vi "2_PatchCore_Inference(Image).vi"() -> ()   [LabVIEW 2020]
uses:
  PatchCore_AddOn/API/Controls/NN_Paths.ctl
  PatchCore_AddOn/API/Controls/PatchCore_Init_Custom_NN_CFG.ctl
  <vilib>/Ngene/Deep Learning Toolkit/Toolkit/NN_Data/API/NN_Dims(C,H,W).ctl
  <vilib>/Ngene/Deep Learning Toolkit/Toolkit/NN_Network/Controls/NN_Device.ctl
  PatchCore_AddOn/API/Controls/Heatmap_Config.ctl
  PatchCore_AddOn/API/Controls/ColorMap.ctl
  PatchCore_AddOn/API/Controls/Feature_Scorer_Params.ctl
  PatchCore_AddOn/API/Controls/Gaussian_Blur.ctl
  PatchCore_AddOn/API/Controls/PCore_Device.ctl
  <vilib>/Utility/miscctls.llb/LVMinMaxIncTypeDef.ctl
  subVIs/Dataset_Reader/Controls/ImRead_PreProcessing_Options.ctl
  PatchCore_AddOn/Low_Level/Controls/Normalization_Type.ctl
  PatchCore_AddOn/API/NNPC_Predict/NNPC_Predict(Single).vi
  PatchCore_AddOn/PatchCore_AddOn.lvlib
  <vilib>/Ngene/Deep Learning Toolkit/Toolkit/Deep_Learning_Toolkit_by_Ngene.lvlib
panel:
  in  "PCore_Device":T1=enum."GPU(CuLab)"
  out "Image_Thrshld (Eval)":sgl=1.3846
  in  "Image_Thrshld(Custom)":sgl=-1.0 format="%_5g"
  out "dT_Predict":dbl=0.00989810000001512 format="%#_3ps"
  out "Pixel_Score(Min)":sgl=0.030176789
  out "Pixel_Score(Max)":sgl=2.5852501
  out "Image_File_Path":path=path "D:/MVTec/bottle/test/broken_large/011.png"
  in  "Feature_Scorer_Params":T2={"Nearest_Neihbours"=1, "Calculate Anomaly Map"=TRUE, "Gaussian_Blur"={"Kernel_Size"=33, "sigma"=4.0}}
  out "Pixel_Thrshld (Eval)":sgl=1.2317
  in  "Report_Image_Dims":cluster{"X Resolution":i32, "Y Resolution":i32}={"X Resolution"=224, "Y Resolution"=224}
  in  "Stop":bool
  in  "Heatmap_Config":T4={"ColorMap_Type"=enum."Jet", "Alpha"=0.4}
  out "Anomaly?":bool=TRUE
  in  "Eval_Stats_File_Path":path=path "D:/Ngene/GitHub/3_Image_Processing/36_Anomaly_Detection/Models/Patchcore_Models/__24_10_30__20_44_16/PatchCore_Eval_Stats__24_10_30__20_47_45.cfg"
  out "dT_ImRead":dbl=0.02204290000000242 format="%#_4ps"
  in  "NNFE_Custom_CFG":T6={"Input3D_Custom_Dims"={"C"=-1, "H"=-1, "W"=-1}, "mBatch"=1, "NN_Device"=enum."GPU"}
  in  "PatchCore_Paths":T9={"CFG"=path "D:/Ngene/GitHub/3_Image_Processing/36_Anomaly_Detection/Models/Patchcore_Models/__24_10_30__20_44_16/PatchCore_Config.cfg", "BIN"=path "D:/Ngene/GitHub/3_Image_Processing/36_Anomaly_Detection/Models/Patchcore_Models/__24_10_30__20_44_16/MemBank_NNFE_WRN_50_2_L2L3_PS3_RP296_SR0.1_Size16.4k.bin"}
  in  "NNFE_Paths":T9={"CFG"=path "D:/Ngene/GitHub/3_Image_Processing/36_Anomaly_Detection/Models/Patchcore_Models/__24_10_30__20_44_16/NNFE_WRN_50_2_L2L3_PS3_RP296.cfg", "BIN"=path "D:/Ngene/GitHub/3_Image_Processing/36_Anomaly_Detection/Models/Patchcore_Models/__24_10_30__20_44_16/NNFE_WRN_50_2_L2L3_PS3_RP296.bin"}
  out "Anomaly Detection Results":T10(plugin-control)
  out "Img_Score":sgl=2.7060041
  in  "Image_idx":u32=31 max=82
  in  "Ground_Truth_Folder_Path":path=path "D:/MVTec/bottle/ground_truth"
  in  "Pixel_Thrshld(Custom)":sgl=-1.0 format="%_5g"
  in  "Test_Dataset_Folder_Path":path=path "D:/MVTec/bottle/test"
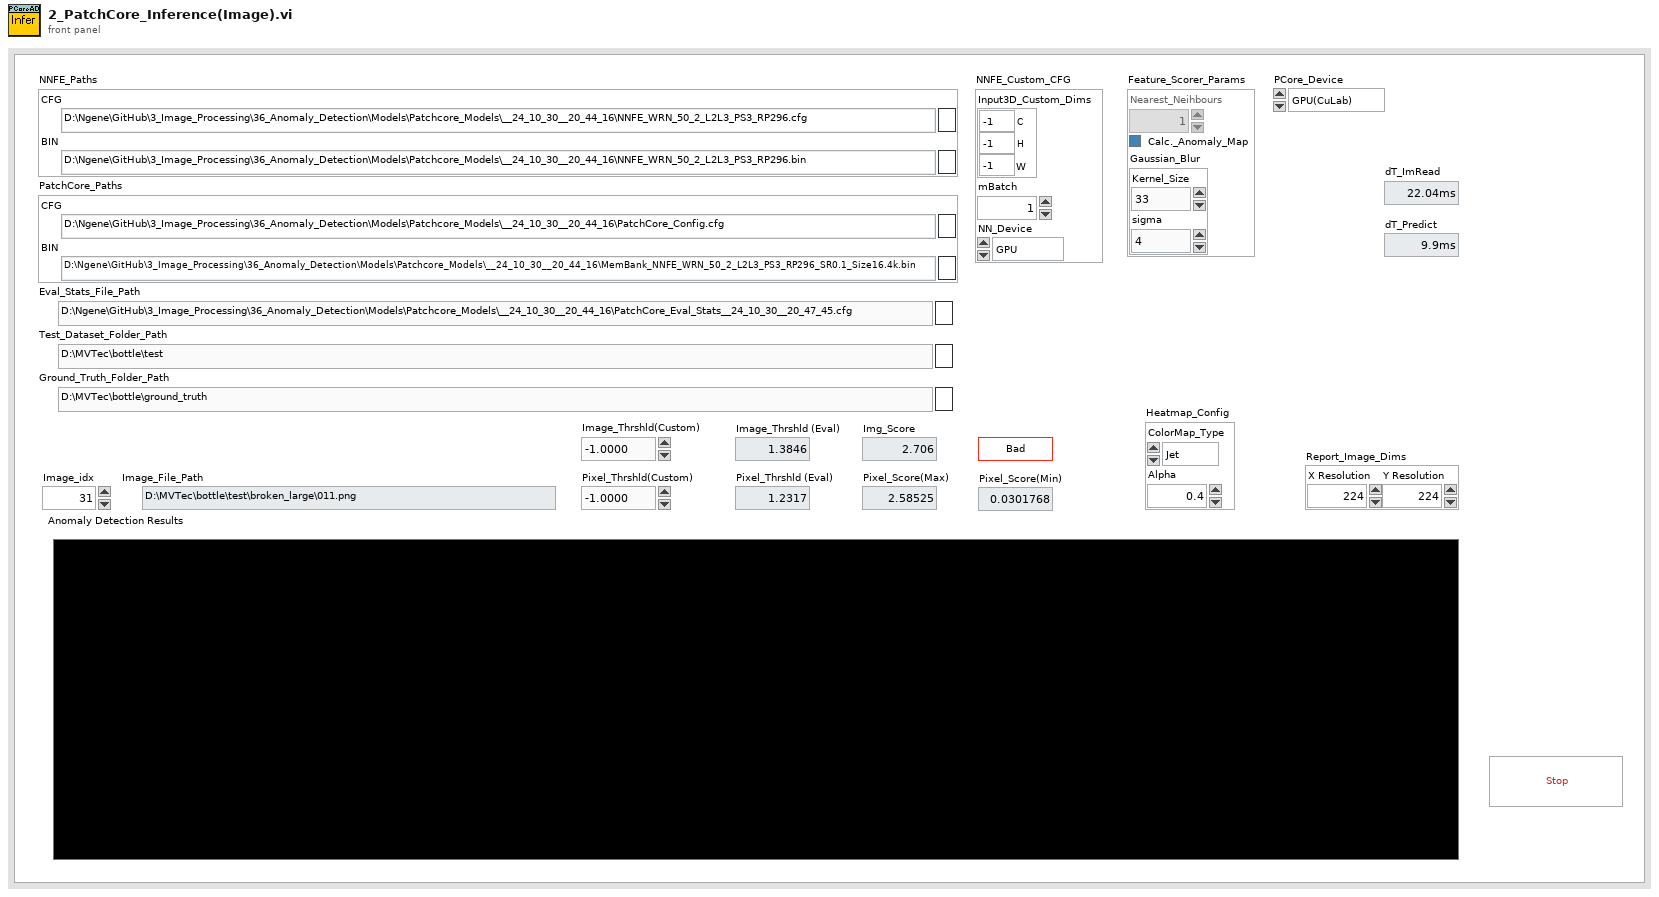
[diagram p1: front panel]
types:
  T1 = typedef "PatchCore_AddOn.lvlib/PCore_Device.ctl" = enum16{"CPU", "GPU(CuLab)"}
  T2 = typedef "PatchCore_AddOn.lvlib/Feature_Scorer_Params.ctl" = cluster{"Nearest_Neihbours":i32, "Calculate Anomaly Map":bool, "Gaussian_Blur":T3}
  T3 = typedef "PatchCore_AddOn.lvlib/Gaussian_Blur.ctl" = cluster{"Kernel_Size":i32, "sigma":sgl}
  T4 = typedef "PatchCore_AddOn.lvlib/Heatmap_Config.ctl" = cluster{"ColorMap_Type":T5, "Alpha":sgl}
  T5 = typedef "PatchCore_AddOn.lvlib/ColorMap.ctl" = enum16{"Jet", "Perula", "Inferno", "Plasma", "Viridis"}
  T6 = typedef "PatchCore_AddOn.lvlib/PatchCore_Init_Custom_NN_CFG.ctl" = cluster{"Input3D_Custom_Dims":T7, "mBatch":i32, "NN_Device":T8}
  T7 = typedef "Deep_Learning_Toolkit_by_Ngene.lvlib/NN_Dims(C,H,W).ctl" = cluster{"C":i32, "H":i32, "W":i32}
  T8 = typedef "Deep_Learning_Toolkit_by_Ngene.lvlib/NN_Device.ctl" = enum16{"CPU", "GPU"}
  T9 = typedef "PatchCore_AddOn.lvlib/NN_Paths.ctl" = cluster{"CFG":path, "BIN":path}
  T10 = typedef "IMAQ Image.ctl" = refnum<image>
  T11 = typedef "LVMinMaxIncTypeDef.ctl" = cluster{"Minimum":dbl, "Maximum":dbl, "Increment":dbl}
  T12 = typedef "PatchCore_AddOn.lvlib/PatchCore_Instance.ctl" = cluster{"Dataset_Stats":T13, "NN":T15, "PCore_Device":T1, "PatchCore_Init_CFG":T30, "Coreset Params":T32, "MemBank_Data":T34}
  T13 = typedef "PatchCore_AddOn.lvlib/PatchCore_DS_Stats.ctl" = cluster{"means":T14, "vars":T14, "DS_Size":i32}
  T14 = typedef "PatchCore_AddOn.lvlib/Image_Stats_RGB.ctl" = cluster{"R":sgl, "G":sgl, "B":sgl}
  T15 = typedef "Deep_Learning_Toolkit_by_Ngene.lvlib/NN.ctl" = cluster{"Name":string, "No of Layers":i32, "mBatch":i32, "Layers":T16[], "Dimty":T17, "Dims_In":T7, "Dims_Out":T7, "Working_Dir":path, "Train?":bool, "Train_Params":T18, "LR_Update_Policy":T21, "Session Data":T23, "Ground_truth":T24, "NNg_hdls":T25, "NN_Device":T8, "GPU Id":i32, "Labels":string[], "Receptive Field":T26[], "Loss_Type":T27, "Loss_Cfg_Prms":variant, "NNG_WS":T28}
  T16 = typedef "Deep_Learning_Toolkit_by_Ngene.lvlib/NN_Layer_ref.ctl" = refnum<data-value>
  T17 = typedef "Deep_Learning_Toolkit_by_Ngene.lvlib/NN_In_Out_Dim-ty.ctl" = enum8{"In1D_Out1D", "In3D_Out1D", "In3D_Out3D", "In3D_OutBBox"}
  T18 = typedef "Deep_Learning_Toolkit_by_Ngene.lvlib/NN_Train_Params.ctl" = cluster{"Optimizer":T19, "Beta_1":sgl, "Beta_2":sgl, "Weight Decay(L1)":sgl, "Weight Decay(L2)":sgl, "Data_Sampling":T20}
  T19 = typedef "Deep_Learning_Toolkit_by_Ngene.lvlib/NN_Train_Optimizer.ctl" = enum16{"SGD", "Adam", "Adagrad", "Adadelta", "RMSProp", "Nesterov"}
  T20 = typedef "Deep_Learning_Toolkit_by_Ngene.lvlib/NN_Train_Data_Sampling.ctl" = enum16{"Random", "Sequential"}
  T21 = typedef "Deep_Learning_Toolkit_by_Ngene.lvlib/NN_LR_Policy_Cfg.ctl" = cluster{"Policy_Type":T22, "LR0":dbl, "k":sgl, "WarmUp_Policy":enum16{"Step", "Ramp"}, "WarmUp_Iter":i32, "WarmUp_Ratio":sgl}
  T22 = typedef "Deep_Learning_Toolkit_by_Ngene.lvlib/NN_LR_Policy_Type.ctl" = enum16{"Manual", "Step", "Exp", "1/t"}
  T23 = typedef "Deep_Learning_Toolkit_by_Ngene.lvlib/NN_Train_Session_Data.ctl" = cluster{"Epochs":sgl, "Tot_Iter":i32, "LR":sgl, "LR_iter":i32}
  T24 = typedef "Deep_Learning_Toolkit_by_Ngene.lvlib/NN_Ground_truth.ctl" = cluster{"Y":variant}
  T25 = typedef "Deep_Learning_Toolkit_by_Ngene.lvlib/nng_cuda_handles.ctl" = cluster{"cudnn":u64, "cublas":u64, "stream":u64, "curand":u64}
  T26 = typedef "Deep_Learning_Toolkit_by_Ngene.lvlib/NN_Dims(V,H).ctl" = cluster{"V":i32, "H":i32}
  T27 = typedef "Deep_Learning_Toolkit_by_Ngene.lvlib/NN_Loss_Type.ctl" = enum16{"None", "MSE", "CrossEntropy", "YOLO_v2", "YOLO_v4"}
  T28 = typedef "Deep_Learning_Toolkit_by_Ngene.lvlib/NNG_WS.ctl" = cluster{"NNG_WS_Mem":T29, "Max_WS_Size":i64}
  T29 = typedef "Deep_Learning_Toolkit_by_Ngene.lvlib/NNg_WS_Mem_DVR.ctl" = refnum<data-value>
  T30 = typedef "PatchCore_AddOn.lvlib/PatchCore_Init_CFG.ctl" = cluster{"BackBone":T31, "Out_Layers_Names":string[], "Patch_Size":u32}
  T31 = typedef "PatchCore_AddOn.lvlib/PatchCore_BackBone_Selector.ctl" = enum16{"WRN_50_2_L2L3"}
  T32 = typedef "PatchCore_AddOn.lvlib/Coreset_Params.ctl" = cluster{"Sampling_Ratio":sgl, "Startd_idx":i32, "Random_Proj?":bool, "Rnd. Proj. Params":T33}
  T33 = typedef "PatchCore_AddOn.lvlib/Random_Projection_Coreset.ctl" = cluster{"Proj._Dim.":i32, "Epsilon":sgl, "Seed":i32}
  T34 = typedef "PatchCore_AddOn.lvlib/MemBank_and_Norm_Variants.ctl" = cluster{"MemBank":variant, "MemBank Norm":variant}
  T35 = typedef "PatchCore_AddOn.lvlib/Eval_Results.ctl" = cluster{"Scores(Good)":T36, "Scores(Bad)":T36, "F1_Max":sgl, "Thrshld(F1_Max)":sgl, "IoU_Max":sgl, "Thrshld(IoU_Max)":sgl, "AUROC":sgl}
  T36 = typedef "PatchCore_AddOn.lvlib/MinMax.ctl" = cluster{"Min":sgl, "Max":sgl}
  T37 = typedef "ImRead_PreProcessing_Options.ctl" = cluster{"Image Type":T38, "Normalization Type":T39, "Interpolation Type":u32}
  T38 = typedef "Image Type" = u32
  T39 = typedef "PatchCore_AddOn.lvlib/Normalization_Type.ctl" = enum16{"Standardize(DS_Stats)", "Standardize(Image_Stats)"}
  T40 = typedef "PatchCore_AddOn.lvlib/Anomaly_Detection_Results_Imgs.ctl" = cluster{"Image":T10, "Ground Truth":T10, "Predicted Heat Map":T10, "Predicted Mask":T10, "Segmentation":T10}
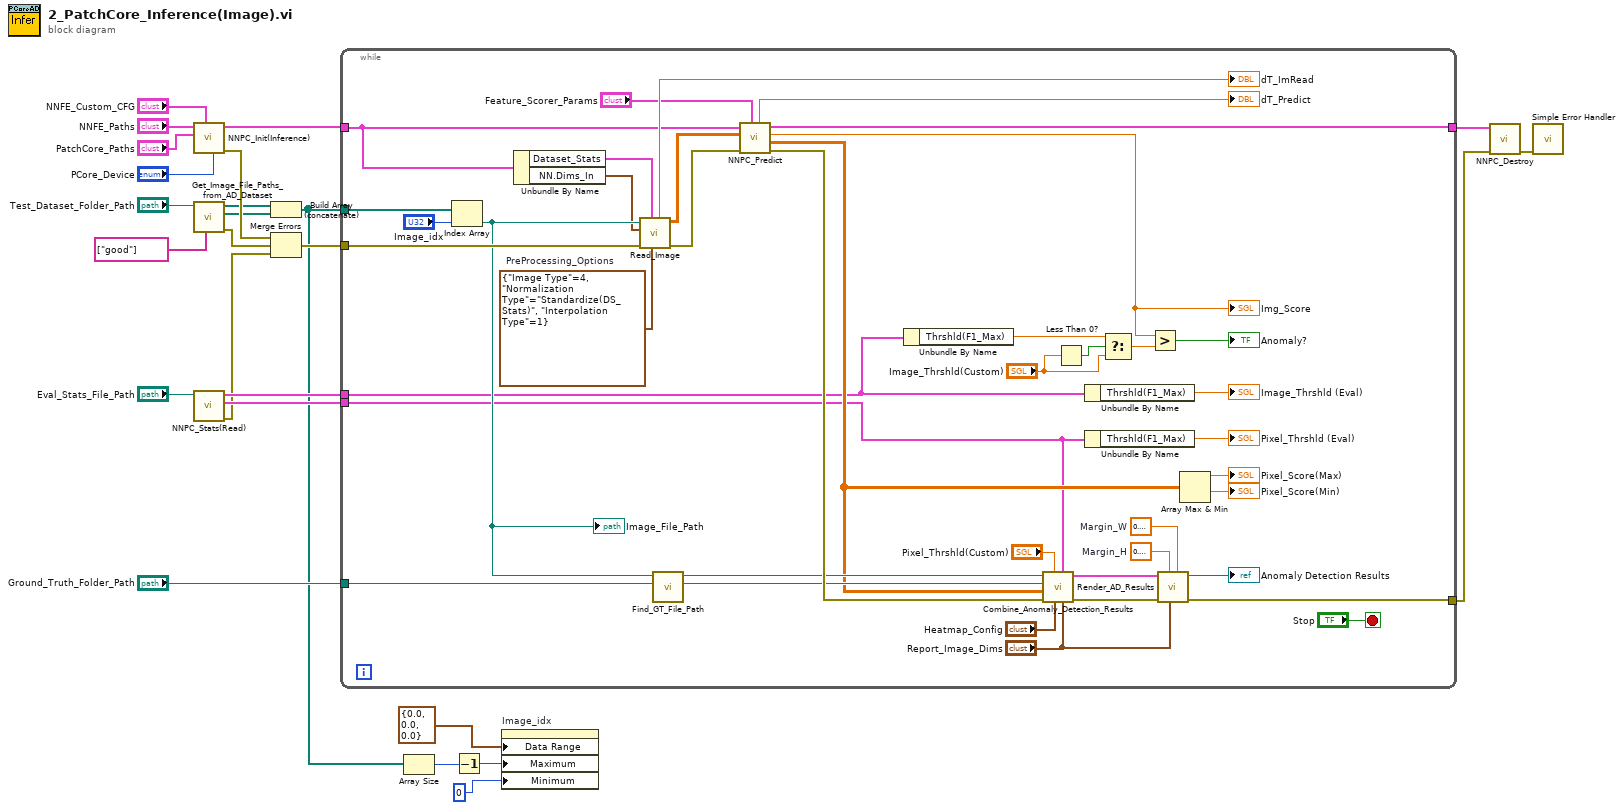
[diagram p0: block diagram]
diagram:
  n1 = call "NNPC_Init(Inference).vi"("PCore_Device"="PCore_Device", "NNFE_Custom_CFG"="NNFE_Custom_CFG", "PatchCore_Paths"="PatchCore_Paths", "NNFE_Paths"="NNFE_Paths") -> ("error out"=w14:errorcluster, "PCore_Instance out"=w19:T12)  [unwired: 6 in]
  n2 = call "Get_Image_File_Paths_from_AD_Dataset.vi"("Good Folder Names"=string[] ["good"] ("Good Folder Name"), "Dataset Folder"="Test_Dataset_Folder_Path") -> ("error out"=w9:errorcluster, "Bad Dataset Files"=w2:path[], "Good Dataset Files"=w1:path[])  [unwired: 7 in]
  n3 = call "NNPC_Stats(Read).vi"("CFG file path"="Eval_Stats_File_Path") -> ("error out"=w13:errorcluster, "Pixel Results"=w15:T35, "Image Results"=w16:T35)  [unwired: 8 in]
  n4 = Build Array (concatenate)(w1, w2) -> (w10:path[])
  n5 = Merge Errors(w14, w9, w13) -> (w17:errorcluster)
  n6 = while {
    tunnel: w10 -> [w66]
    tunnel: w19 -> [w41]
    tunnel: [w64] -> w7
    tunnel: w16 -> [w33]
    tunnel: w15 -> [w32]
    tunnel: w17 -> [w65]
    tunnel: [w60] -> w8
    tunnel: "Ground_Truth_Folder_Path" -> [w44]
    stop <- "Stop" stop-if-true
    w26 = T37 {"Image Type"=4, "Normalization Type"=enum."Standardize(DS_Stats)", "Interpolation Type"=1}  # PreProcessing_Options
    w54 = sgl 0.2  # Margin_W
    w55 = sgl 0.2  # Margin_H
    n7 = Index Array(array=w66, index="Image_idx") -> (element=w47:path)
    "Image_File_Path" <- w47
    n8 = Unbundle By Name(w41) -> ("Dataset_Stats"=w28:T13, "NN.Dims_In"=w27:T7)
    n9 = call "Read_Image.vi"("PreProcessing_Options"=w26, "Dataset_Stats"=w28, "error in"=w65, "Target_Dims"=w27, "Img Path"=w47) -> ("error out"=w29:errorcluster, "Image Out"=w30:sgl[][][], "dT_Img_Read"=→"dT_ImRead":dbl)  [unwired: 4 in]
    n10 = call "Find_GT_File_Path.vi"("GT Mask Folder Path"=w44, "Image File Path"=w47) -> ("GT File Path"=w45:path, "Image File Path out"=w46:path)  [unwired: 8 in]
    n11 = call-poly "NNPC_Predict.vi"("Feature Scorer Params"="Feature_Scorer_Params", "error in"=w29, "Image in"=w30, "PCore_Instance in"=w41) -> ("error out"=w62:errorcluster, "anomaly map"=w39:sgl[][], "pred score"=w38:sgl, "PCore_Instance out"=w64:T12, "dT_Predict"=→"dT_Predict":dbl)  [unwired: 3 in]
    "Img_Score" <- w38
    n12 = Unbundle By Name(w33) -> ("Thrshld(F1_Max)"=w50:sgl)
    n13 = call "Combine_Anomaly_Detection_Results.vi"("Infrnc Dims"="Report_Image_Dims", "Pixel Results"=w32, "Heatmap Config"="Heatmap_Config", "Pixel Anomaly Thrshld"="Pixel_Thrshld(Custom)", "error in"=w62, "Anomaly Map"=w39, "Gt File Path"=w45, "Img File Path"=w46) -> ("error out"=w61:errorcluster, "Anomaly Detection Rresults"=w59:T40)  [unwired: 1 in, 1 out]
    n14 = Less Than 0?(x="Image_Thrshld(Custom)") -> (x < 0?=w52:bool)
    n15 = Unbundle By Name(w33) -> ("Thrshld(F1_Max)"=→"Image_Thrshld (Eval)":sgl)
    n16 = Unbundle By Name(w32) -> ("Thrshld(F1_Max)"=→"Pixel_Thrshld (Eval)":sgl)
    n17 = Select(t=w50, s=w52, f="Image_Thrshld(Custom)") -> (s? t:f=w49:sgl)
    n18 = Greater?(x=w38, y=w49) -> (0:→"Anomaly?":bool)
    n19 = call "Render_AD_Results.vi"("Margin_W"=w54, "Image_Dims"="Report_Image_Dims", "Margin_H"=w55, "error in"=w61, "Anomaly Detection Rresults"=w59) -> ("error out"=w60:errorcluster, "Anomaly Detection Results"=→"Anomaly Detection Results":T10)  [unwired: 5 in]
    n20 = Array Max & Min(array=w39) -> (max value=→"Pixel_Score(Max)":sgl, min value=→"Pixel_Score(Min)":sgl)  [unwired: 2 out]
  }
  n21 = Array Size(array=w10) -> (size(s)=w25:i32)
  n22 = Decrement(x=w25) -> (x-1=w24:i32)
  n23 = property on="Image_idx" class="DigNum (strict)"("Data Range"=T11 {"Minimum"=0.0, "Maximum"=0.0, "Increment"=0.0} ("Data Entry Limits"), "Maximum"=w24, "Minimum"=u32 0 ("Data Entry Limits:Minimum")) -> ()  [unwired: 2 in, 2 out]
  n24 = call "NNPC_Destroy.vi"("error in"=w8, "PCore_Instance in"=w7) -> ("error out"=w6:errorcluster)  [unwired: 9 in]
  n25 = call <vilib>:"Simple Error Handler.vi"("error in (no error)"=w6) -> ()  [unwired: 4 in, 5 out]
